vi "MCL Wfma Setup.vi"(0 "wfDacX":dbl, 1 "milliseconds":dbl, 2 "handle":i32, 5 "wfDacY":dbl, 7 "wfDacZ":dbl, 9 "dataPointsPerAxis":i32, 12 "iterations":u16) -> (4 "wfDacX out":dbl, 6 "wfDacY out":dbl, 8 "wfDacZ out":dbl, 10 "function return":i32)   [LabVIEW 2017, in "Madlib.lvlib"]
doc: "MADLIB_API int MCL_WfmaSetup(double *wfDacX, double *wfDacY, double *wfDacZ, int dataPointsPerAxis, double milliseconds, unsigned short iterations, int handle);"
uses:
  Madlib.lvlib
  Madlib.dll
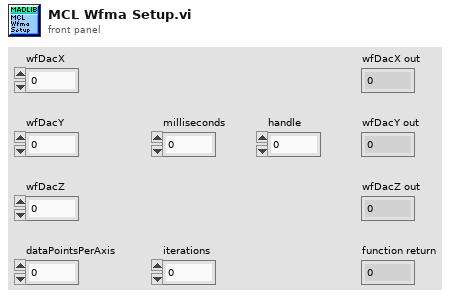
[diagram p1: front panel]
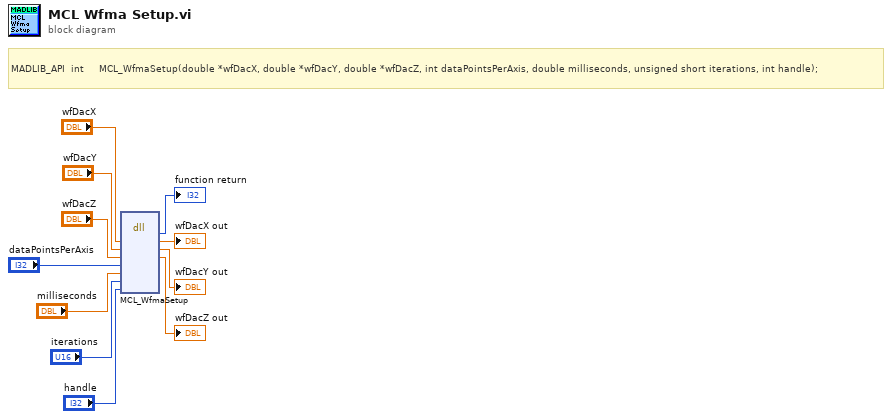
[diagram p0: block diagram]
diagram:
  # "MADLIB_API  int     MCL_WfmaSetup(double *wfDacX, double *wfDacY, double *wfDacZ, int dataPointsPerAxis, double milliseconds, unsigned short iterations, int handle);"
  n1 = dll-call lib="C:/Users/francesco/dev/pump-probe/Piezo/lvlib/Madlib.*" fn="MCL_WfmaSetup"("wfDacX"="wfDacX", "wfDacY"="wfDacY", "wfDacZ"="wfDacZ", "dataPointsPerAxis"="dataPointsPerAxis", "milliseconds"="milliseconds", "iterations"="iterations", "handle"="handle") -> (→"function return":i32, "wfDacX"=→"wfDacX out":dbl, "wfDacY"=→"wfDacY out":dbl, "wfDacZ"=→"wfDacZ out":dbl)  [unwired: 7 in, 2 out]
